vi "Table to HTML.vi"(1 "Table":string[][](table)=[["11", "12", "13", "14"], ["21", "22", "23", "24"], ["31", "32", "33", "34"], ["41", "42", "43", "44"]]) -> (0 "HTML-formatted Table":string="<table border=1><tr><td>11</td><td>12</td><td>13</td><td>14</td></tr><tr><td>21</td><td>22</td><td>23</td><td>24</td></tr><tr><td>31</td><td>32</td><td>33</td><td>34</td></tr><tr><td>41</td><td>42</td><td>43</td><td>44</td></tr></table>")   [LabVIEW 2010]
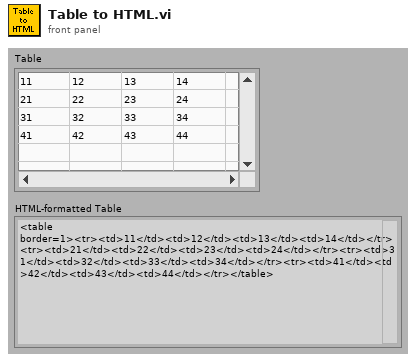
[diagram p1: front panel]
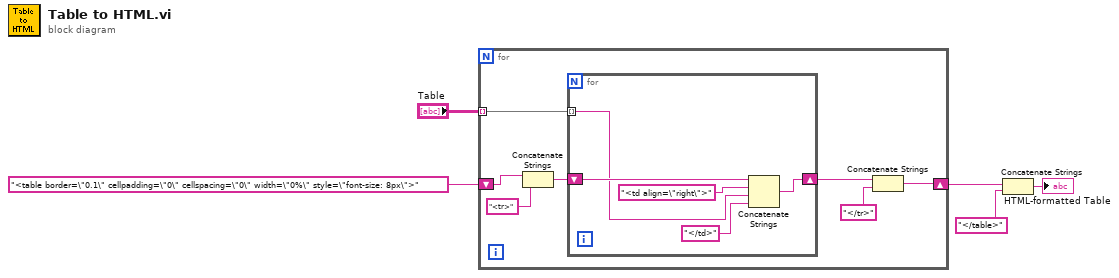
[diagram p0: block diagram]
diagram:
  n1 = for {
    tunnel: "Table" -> [w9] mode=indexing
    shift-right: [w6] -> w3
    shift-left: "<table border=\"0.1\" cellpadding=\"0\" cellspacing=\"0\" width=\"0%\" style=\"font-size: 8px\">" -> [w12]
    n2 = Concatenate Strings(w12, "<tr>" ("string")) -> (w10:string)
    n3 = for {
      shift-right: [w15] -> w8
      shift-left: w10 -> [w16]
      tunnel: w9 -> [w14] mode=indexing
      n4 = Concatenate Strings(w16, "<td align=\"right\">" ("string"), w14, "</td>" ("string")) -> (w15:string)
    }
    n5 = Concatenate Strings(w8, "</tr>" ("string")) -> (w6:string)
  }
  n6 = Concatenate Strings(w3, "</table>" ("string")) -> (→"HTML-formatted Table":string)
